vi "Version_2.0_Single_Column_Code.vi"() -> ()   [LabVIEW 2020]
uses:
  C:/Users/Admin/Desktop/MicroPurification/Developer/MainLabViewProject_V2.0/Thorlabs/Thorlabs.MotionControl.Controls.dll
  MainLabViewProject_V2.0/Thorlabs/Thorlabs.MotionControl.Controls.dll
  C:/Users/Admin/Desktop/MicroPurification/Developer/MainLabViewProject_V2.0/Thorlabs/Thorlabs.MotionControl.KCube.InertialMotorCLI.dll
  MainLabViewProject_V2.0/Thorlabs/Thorlabs.MotionControl.KCube.InertialMotorCLI.dll
  <vilib>/Instr/_visa.llb/VISA Configure Serial Port (Instr).vi
  <vilib>/Waveform/WDTOps.llb/WDT Append Waveforms DBL.vi
  <vilib>/Fluigent/Fluigent SDK/sourceCode/fgt_SDK.lvlib
panel:
  in  "n1":dbl=2.0
  in  "Set - Blotting Time":bool
  in  "Set - Blotting Angle":bool
  in  "Automated Blotting \nand Plunging":bool=TRUE
  in  "Blotting Time":dbl=1000.0
  in  "Blotting Angle":dbl=10.0
  in  "Amount of \nGrid Shift \nfor Blotting (um)":i32
  out "Ethane Temperature":dbl
  out "RH (%)":dbl
  out "Valve Closing \nPressure Measured":sgl
  out "Suction pressure \nmeasured":sgl
  in  "Divert Elution Buffer\ninto Column-1":bool
  in  "Discard volume \npriot to elution":dbl=1.0
  in  "Buffer-B Dispense\nFlow Rate for Elution \ntubing pre-wash":dbl=2.0
  in  "Buffer-B Volume \nfor elution tubing \npre-wash":dbl=20.0
  in  "External Valve \nOpen":bool
  in  "N-B1":i32=4
  in  "Valve V10 Open":bool=TRUE
  in  "Valve V9 Open":bool=TRUE
  in  "Valve V8 Open":bool=TRUE
  in  "Capillary purge \nvolume after every\ngrid plunging":dbl=0.05
  in  "Automatic purging \nof capillary after \ngrid deposition":bool=TRUE
  in  "No. of \ncleaning cycles":i32=4
  in  "Pause Elution\nValue":dbl
  in  "Re-SEC":bool
  in  "Buffer-C2 Dispense \nFlow Rate for Washing \nPrior to re-introducing Sample":dbl=2.0
  in  "Buffer-C2 \nWash Volume\nPrior to re-introducing \nSample":dbl=20.0
  in  "Wash column-2 Prior \nto re-introducing \nsample":bool=TRUE
  in  "Valve V7 Open":bool=TRUE
  in  "Valve V6 Open":bool=TRUE
  in  "Valve V5 Open":bool=TRUE
  in  "Fluigent\nLink S/N":u16=10704
  in  "Move Grid \nDown Faster":dbl
  in  "Move Grid \nUp Faster":dbl
  in  "Affinity Elution \nGraph Min CutOff":dbl=1.0
  out "Affinity Elution \nis Approaching":bool
  out "Elution of Column-2":bool
  in  "Port for \nC2-Elution":string="5"
  out "Elution of Column-1":bool
  in  "Port for \nB-Elution":string="7"
  in  "f":dbl
  out "Washing Column-2":bool
  out "Washing Column-1":bool
  in  "Port for \nA2-Wash":string="4"
  out "Sample pumping \ninto Column-1":bool
  out "Equilibriating \nColumn-2":bool
  out "Equilibriating \nColumn-1":bool
  in  "V-S":dbl=10.0
  in  "Port for \nSample":string="3"
  in  "N-S":i32=1
  in  "External Valve \nCLOSED":string="2"
  in  "External Valve \nOPEN":string="1"
  in  "Port for \nC1-Equilibriation":string="5"
  in  "Port for \nA1-Equilibriation":string="4"
  in  "Port-<n> to be \nCleaned (4-9)":i32(ring) items=["4", "5", "6", "7", "8", "9"]
  in  "Clean the \nBuffer-C2 tubing":bool
  in  "Clean the \nBuffer-B tubing":bool=TRUE
  in  "Signal":bool
  out "Net Elution \nVolume":dbl
  out "Pause Elution":bool
  in  "Apparent Volume\nof Syringe":dbl=20.0
  in  "N-C1":i32=4
  in  "N-A1":i32=4
  in  "On-Chip Valve \nClosing\nPressure (mbar)":dbl=1200.0
  in  "Wait time for\ntranslation":u32=100
  out "Suction pressure \nfor grid deposition":sgl
  in  "Suction Pressure\nfor EM-grid \nDeposition (mbar)":sgl
  out "Amplified Signal with Fluid Volume for Affinity Elution":cluster{"Array":dbl[], "Array":dbl[]}(graph)
  out "Affinity Elution On":bool
  out "Amplified Signal with Fluid Volume Near Affinity Elution":cluster{"Array":dbl[], "Array":dbl[]}(graph)
  in  "Valve V4 Open":bool=TRUE
  out "Affinity On":bool
  out "Amplified Signal with Fluid Volume for SEC":cluster{"Array":dbl[], "Array":dbl[]}(graph)
  out "SEC On":bool
  in  "n":i32
  in  "c":dbl
  in  "Duration for \nup/down\nMovement of Grid":u32=100
  in  "Wait time before \nsolenoid for V2\nturns on 2":u32
  in  "Discard Volume":dbl
  out "Discard fluid \nprior to 1st \ndeposition":bool
  in  "Grid Deposition\nDuration":u32
  in  "Valve V3 Open":bool=TRUE
  in  "Valve V2 Open":bool=TRUE
  in  "Valve V1 Open":bool=TRUE
  in  "Delay before\n1st movement\nof grid":dbl
  in  "No of cycles\nof up-down\nmovement":dbl=7.0
  in  "Translation Step SIze\nwhile plunging":dbl=400.0
  in  "Move\nGrid Down":dbl
  in  "Move\nGrid Up":dbl
  in  "k2":dbl
  in  "k1":dbl
  in  "KCubeInertialMotorControl":refnum<k24>(container)
  in  "Select the Action":T1(ring)
  out "Temperature of Ethane Graph":waveform(dbl)(graph)
  in  "Position":i32
  out "True Volume being \ninjected in this\nprocess":dbl
  in  "Buffer-C Volume \nto be Pumped for\nColumn \nnon-interference":dbl
  in  "Buffer-C1 Dispense\nFlow Rate (ul/min) \nfor Equilibration\nof Column-2":dbl=2.0
  in  "Buffer-C1 Volume \nto be  Pumped \nfor Equilibration\nof Column-2":dbl=55.0
  in  "Buffer-C1 Pumping\nResolution \nfor Equilibration \nof Column-2":T2(ring)=enum."High Resolution Pumping"
  in  "Buffer-C1 PickUp \nFlow Rate (ul/min)\nfor Equilibration \nof Column-2":dbl=150.0
  in  "Buffer-A1 Dispense\nFlow Rate (ul/min) \nfor Equilibration\nof Column-1":dbl=2.0
  in  "Buffer-A1 Volume \nto be  Pumped \nfor Equilibration\nof Column-1":dbl=35.0
  in  "Buffer-A1 Pumping\nResolution \nfor Equilibration \nof Column-1":T2(ring)=enum."High Resolution Pumping"
  in  "Buffer-A1 PickUp \nFlow Rate (ul/min)\nfor Equilibration \nof Column-1":dbl=150.0
  out "Buffer-C Volume\nleft to be Pumped":dbl
  in  "Re-deposit Sample\nonto Grid":bool
  in  "Suction On/Off":bool
  out "Vol_previous":dbl
  out "Vol_now":dbl
  out "Position\nNow":dbl
  out "Sample Volume Diverted\ninto Column-2":dbl
  out "Reminder of the \nVolume to be \nPumped":dbl
  in  "Divert Buffer-C \ninto Column-2":bool=TRUE
  in  "Divert Sample \ninto Column-2":bool
  in  "Buffer-B Volume \nto be Pumped for\nSample Diversion\nto Column-2":dbl=0.5
  out "Amplified Signal with Fluid Volume":cluster{"Array":dbl[], "Array":dbl[]}(graph)
  in  "Stop for End of \nExperiment \nand Data Writing":bool
  in  "Select a Process":T3(ring)
  out "Initial Plunger Position":dbl
  out "Stopper that ends \nthe main loops":bool
  in  "Pause /Continue":bool
  in  "Start the Process":bool
  out "Pause Data Collection":bool
  out "Volume being Injected \ntill the end of previous \nprocess":dbl
  out "Total Volume \nbeing Injected":dbl
  out "Volume being Injected \nin this process":dbl
  in  "Divert Sample \nonto Grid":bool=TRUE
  in  "VISA Refnum in\nfor Valve":refnum<visa-resource-name>="COM3"
  in  "Buffer-C2 Dispense\nFlow Rate (ul/min)":dbl=0.25
  in  "Buffer-C2 Volume \nto be Pumped":dbl
  in  "Buffer-C2 Pumping\nResolution":T2(ring)=enum."High Resolution Pumping"
  in  "Buffer-C2 PickUp \nFlow Rate (ul/min)":dbl=150.0
  in  "Buffer-B Dispense\nFlow Rate (ul/min)":dbl=0.25
  in  "Buffer-B Volume \nto be  Pumped":dbl
  in  "Buffer-B Pumping\nResolution":T2(ring)=enum."High Resolution Pumping"
  in  "Buffer-B PickUp \nFlow Rate (ul/min)":dbl=150.0
  in  "Sample Dispense\nFlow Rate (ul/min)":dbl=2.0
  in  "Sample Volume \nto be Pumped":dbl
  in  "Sample Pumping\nResolution":T2(ring)=enum."High Resolution Pumping"
  in  "Sample PickUp \nFlow Rate (ul/min)":dbl=15.0
  in  "Buffer-A2 Dispense\nFlow Rate (ul/min)":dbl=2.0
  in  "Buffer-A2 Volume \nto be Pumped":dbl
  in  "Buffer-A2 Pumping\nResolution":T2(ring)=enum."High Resolution Pumping"
  in  "Buffer-A2 PickUp \nFlow Rate (ul/min)":dbl=150.0
  in  "Volume of Syringe":dbl=25.0
  in  "VISA Refnum in\nfor Pump":refnum<visa-resource-name>="COM4"
  # "More Notes:\n\n- At the start of the experiment, ensure the extrenal valve is detected by teh program\\\n            - Manually unplug and replug the power connection to the valve (locatd near the valve)\n            - Start the program and click on 'Initialize only the valve\" and click on \"Start the Process\"\n            \n\n              - If the program doesn't initialize the valve in 30 sec, turn off the program.\n             -  Manually unplug and replug the power connection to the valve (locatd near the valve) again\n             - Start the LSPone quick softwar on teh desktop and click on the Mnual setting\n             - Choose 'COM3'\n             - Click on Initialize. If teh initialization is sucessful, close this isftware and turn on the \n                 Labview program and try to inialize teh valve. If the valve gets initialized, you are \n                  good to go and use the program further, else redo the process.\n\n- After the above step, while cleaning the tubings\n             - First cleaning ttubings using IPA ....The code is 'clean tubings 3,4, 5and 7\n             - Clean the tubing that goes to teh chip affinity column twice using IPA, run Buffer-A2 pumping code\n             - Clean the tubing that goes to teh chip SEC column twice using IPA, run Buffer-C2 pumping code\n              - Run the above 3 steps with IPA again. This ensures we have teh least bubbles in teh sysetm\n              - Run the 1st 3 steps with water.\n              - After inserting the tubings to the chip, clean teh affinity and SEC columns at 2 ul/min of 30 ul each with water\n              - Before teh start of the main experimnet, run the  code 'clean the tubing from port-3 vial' with Buffer-A once\n\n               - Place teh sample and all teh buffers in the appropriate places and run teh code  with Re-SEC possibility with \n                  appropriate parameters"
  # "Clean only 3,4,5 and 7 \nfor Complex-I\nunless other ports are used"
  # "Notes specific for this code:\n\n- V1 is teh valve just prior to and after affinity column, all other valves are numbered \nclockwise with valve V8 to be teh valve conncecting affinity inlet to waste outlet-2.\n\n- V9 and V10 are valves for affinity wash and elution inlets. Currently they are not used \nin this code.\n\n- Port-8 is connected to the tubing of elution that is conncetcted to column-1 of chip"
  # "Pump Port No           Function\n         1                       Pump Waste\n         2                       Chip Column-1 Connection\n         3                       Sample\n         4                       Buffer- A1 for Equilibriation of Column-1\n         5                       Buffer- C1 for Equilibriation of Column-2\n         6                       Buffer- A2 for Wash of Column-1\n         7                       Buffer- B for Elution of Column-1\n         8                       Buffer-C2 for Elution of Column-2\n         9                       Buffer- A3 for Wash of Column-1\n        10                      Chip Column-2 Connection"
  # "Column-2 Wash Parameters"
  # "Notes:\n- This code uses USB6002 data acquisition device from NI\n- No PGA and only AD8611ARZ preamp\n- Still uses Arduino Uno and Stepper motor \n- Even though designed for Complex-I, but is more generic\n- The code is meant for a chip with 7-onchip valves that are being \ncontrolled using fluigent P-switch, one external on/off valve\nand the pump with 10 ports\n- The tubings \n            - 0.18 mm ID tubings from port-2 to chip, port-3 to sample vial, \nport-10 to SEC inlet of the chip, port-1 to pump-waste\n             - 0.5 mm ID tubings from port-4 to Buffer-A vial, port-5 to \nBuffer-C vial, and port-7 to Buffer-B vial"
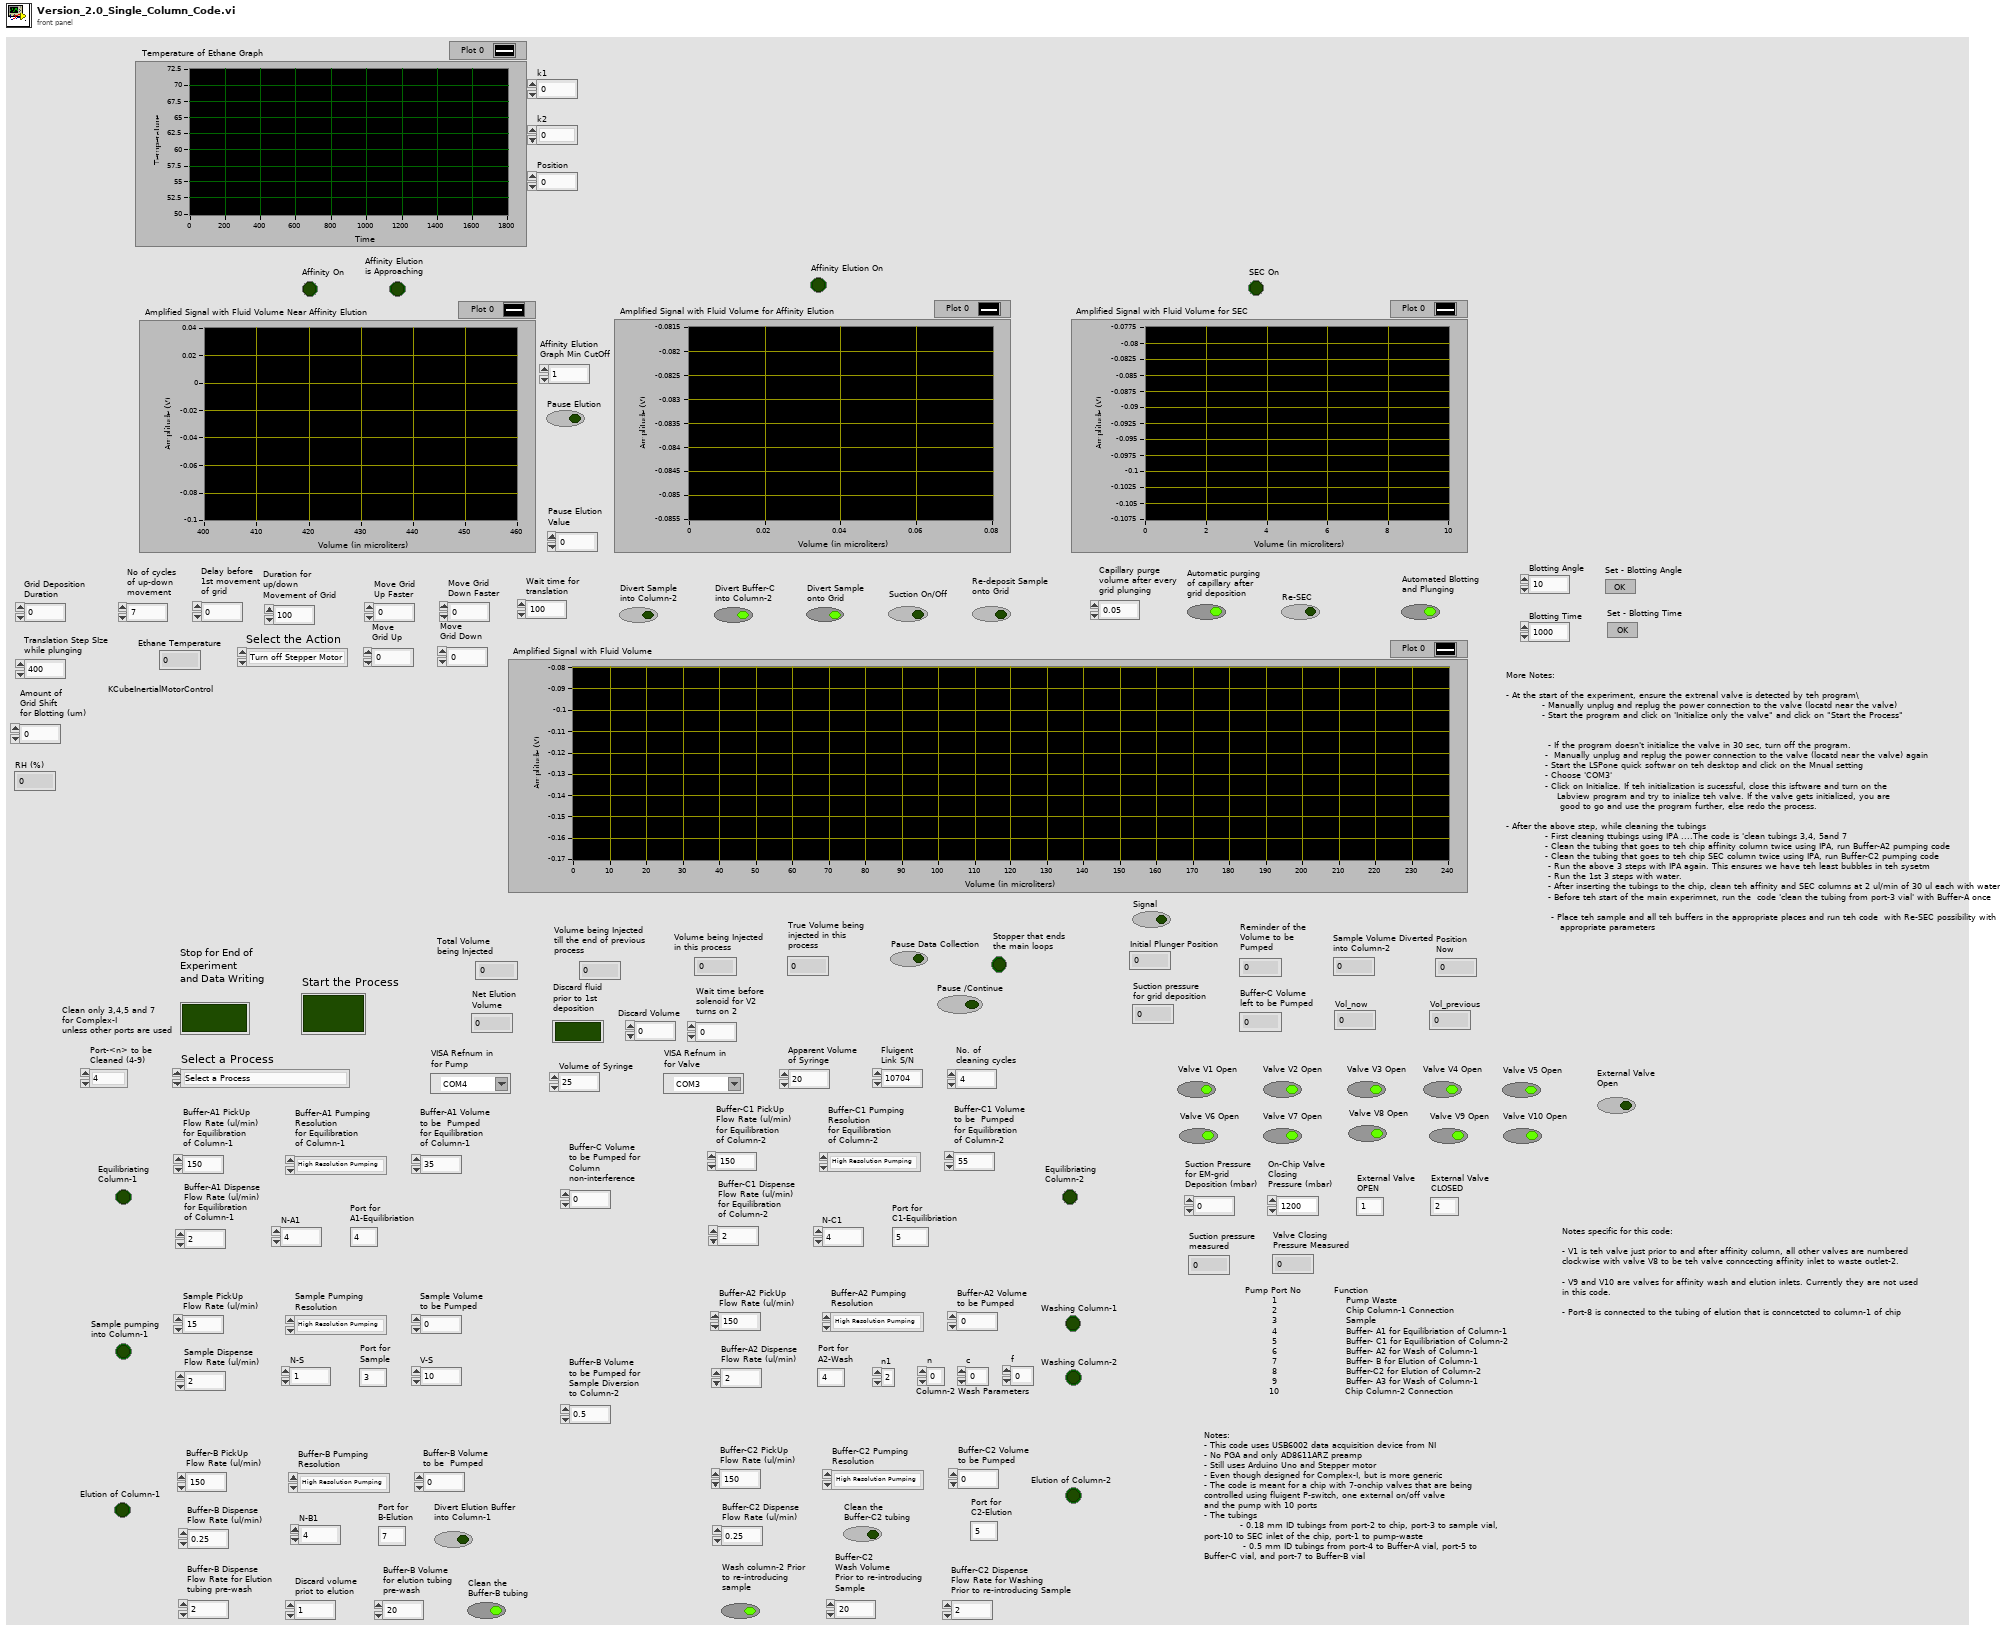
[diagram p1: front panel]
types:
  T1 = enum16{"Turn off Stepper Motor", "Turn  on Stepper Motor", "Spread the deposited protein on the grid in One Line and plunge", "Spread the deposited protein on the grid and plunge", "Start Plunging", "Reset Plunger"}
  T2 = enum16{"Standard Pumping", "High Resolution Pumping"}
  T3 = enum16{"Select a Process", "Initialize Only The Pump", "Initialize Only the Valve", "Initialize Pump and Valve", "Clean the tubing from Port-3 Vial", "Clean the tubing from Port-<n> Vial", "Clean the tubing from Ports 3,4,7 and wash the column", "Clean the tubing from Ports 3,4,5 and 7", "Single Column Automated Protein Purification and Plunging", "Automated Protein Purification with Re-SEC Possibility, 8 SOD Valves and On/Off External Valve", "Automated Protein Purification with 7 SOD Valves and On/Off External Valve", "Automated Plunging Alone Using Purified Protein Via Chip", "Automated Plunging alone using purified protein from SEC column", "Inject Buffer A2, Column 1 with 4 SOD Valves", "Single Column Wash Buffer-A", "Single Column Elution Buffer-B", "Inject Sample, Column 1", "Inject Buffer B, Column 1 with 4 SOD Valves", "Inject Buffer C2, Column 2 with 4 SOD Valves", "Check_Suction_Valve_functionality"}
diagram:
  # "Valve V3 is the on-chip SOD Valve that is after the column-2, after valve V1 and on the way to the waste outlet"
  # "Valve V2 is the on-chip SOD Valve that is after the column-2, after valve V1 and on the way to capillary."
  # "Valve V1 is the on-chip SOD Valve that is after the column-2, just after detection zone-2"
  # "Valve V4 is the on-chip SOD Valve that is after the column-1, just prior to column-2"
  n1 = stacked-sequence {
    frame #0 {
      # "Plunger Control and Ethane Chamber Temperature Display"
      # "AMPLIFIER BLOCK"
      n2 = property class="KCubeInertialMotorControl"(reference="KCubeInertialMotorControl", "SerialNumber"="97102163" ("Serial Number")) -> (reference out=w74:refnum<k24>, error out=w81:errorcluster)  [unwired: 1 in]
      n3 = while {
        stop <- w528 stop-if-true
        n4 = case shown="\"Single Column Automated Protein Purification and Plunging\"" "Select a Process" {
          frame "Initialize Pump and Valve" {
            n5 = local read "Stop for End of \nExperiment \nand Data Writing"() -> (w530:bool)
            n6 = case shown="False" w530 {
              frame False {
                n7 = local read "Start the Process"() -> (w531:bool)
                n8 = case shown="True" w531 {
                  frame False {
                    n9 = local read "Stopper that ends \nthe main loops"() -> (w533:bool)
                    n10 = local read "Start the Process"() -> (w534:bool)
                    n11 = Or(x=w534, y=w533) -> (x .or. y?=w532:bool)
                    n12 = case shown="False" w532 {
                      frame False {
                        n13 = while {
                          stop <- w537 stop-if-true
                          n14 = local read "Stopper that ends \nthe main loops"() -> (w539:bool)
                          n15 = local read "Start the Process"() -> (w538:bool)
                          n16 = Or(x=w538, y=w539) -> (x .or. y?=w537:bool)
                          n17 = Wait (ms)(milliseconds to wait=u32 10) -> ()  [unwired: 1 out]
                        }
                        n18 = One Button Dialog(message="Please select the process and press the 'Start Process' Button") -> ()  [unwired: 1 in, 1 out]
                      }
                      frame True {
                      }
                    }
                  }
                  frame True {
                    n19 = stacked-sequence {
                      frame #0 {
                        n20 = local read "VISA Refnum in\nfor Pump"() -> (w540:refnum<visa-resource-name>)
                        n21 = call "Initializer (SubVI).vi"("VISA Refnum in"=w540) -> ()  [unwired: 11 in]
                      }
                      frame #1 {
                        n22 = local read "VISA Refnum in\nfor Pump"() -> (w541:refnum<visa-resource-name>)
                        n23 = call "ProcessCompletionWaiter (SubVI).vi"("VISA Refnum in"=w541) -> ()  [unwired: 11 in]
                      }
                      frame #2 {
                        n24 = local read "VISA Refnum in\nfor Valve"() -> (w542:refnum<visa-resource-name>)
                        n25 = call "Initializer_Valve (SubVI).vi"("VISA Refnum in"=w542) -> ()  [unwired: 11 in]
                      }
                      frame #3 {
                        n26 = local read "VISA Refnum in\nfor Valve"() -> (w543:refnum<visa-resource-name>)
                        n27 = call "ProcessCompletionWaiter (SubVI).vi"("VISA Refnum in"=w543) -> ()  [unwired: 11 in]
                      }
                      frame #4 {
                        n28 = local write "Start the Process"(FALSE ("Start the Process")) -> ()
                      }
                    }
                  }
                }
              }
              frame True {
              }
            }
          }
          frame "Inject Sample, Column 1" {
            n29 = local read "Stopper that ends \nthe main loops"() -> (w545:bool)
            n30 = case shown="False" w545 {
              frame False {
                n31 = local read "Start the Process"() -> (w546:bool)
                n32 = case shown="True" w546 {
                  frame False {
                    n33 = local read "Stopper that ends \nthe main loops"() -> (w548:bool)
                    n34 = local read "Start the Process"() -> (w547:bool)
                    n35 = Or(x=w548, y=w547) -> (x .or. y?=w549:bool)
                    n36 = case shown="False" w549 {
                      frame False {
                        n37 = while {
                          stop <- w552 stop-if-true
                          n38 = local read "Stopper that ends \nthe main loops"() -> (w554:bool)
                          n39 = local read "Stop for End of \nExperiment \nand Data Writing"() -> (w551:bool)
                          n40 = local read "Start the Process"() -> (w553:bool)
                          n41 = Wait (ms)(milliseconds to wait=u32 10) -> ()  [unwired: 1 out]
                          n42 = Or(x=w554, y=w553) -> (x .or. y?=w552:bool)
                          n43 = local write "Stopper that ends \nthe main loops"(w551) -> ()
                        }
                        n44 = One Button Dialog(message="Please Select the Process and Press 'Start the Process' Button") -> ()  [unwired: 1 in, 1 out]
                      }
                      frame True {
                      }
                    }
                  }
                  frame True {
                    n45 = stacked-sequence {
                      frame #0 {
                        n46 = local read "Sample Volume \nto be Pumped"() -> (w559:dbl)
                        n47 = local read "Apparent Volume\nof Syringe"() -> (w558:dbl)
                        n48 = Quotient & Remainder(x=w559, y=w558) -> (x-y*floor(x/y)=w557:dbl, floor(x/y)=w556:dbl)
                        n49 = for {
                          N: w556 -> [_]
                          n50 = stacked-sequence {
                            frame #0 {
                              # "Switch to Port-3"
                              # "Port-3 of pump is connected to Sample"
                              n51 = local read "VISA Refnum in\nfor Pump"() -> (w561:refnum<visa-resource-name>)
                              n52 = local read "Port for \nSample"() -> (w560:string)
                              n53 = call "PortChanger (SubVI).vi"("Port Number"=w560, "VISA Refnum in"=w561) -> ()  [unwired: 10 in]
                            }
                            frame #1 {
                              n54 = local read "VISA Refnum in\nfor Pump"() -> (w562:refnum<visa-resource-name>)
                              n55 = call "ProcessCompletionWaiter (SubVI).vi"("VISA Refnum in"=w562) -> ()  [unwired: 11 in]
                            }
                            frame #2 {
                              n56 = local read "Sample PickUp \nFlow Rate (ul/min)"() -> (w565:dbl)
                              n57 = local read "Sample Pumping\nResolution"() -> (w564:T2)
                              n58 = local read "VISA Refnum in\nfor Pump"() -> (w567:refnum<visa-resource-name>)
                              n59 = local read "Apparent Volume\nof Syringe"() -> (w563:dbl)
                              n60 = local read "Volume of Syringe"() -> (w566:dbl)
                              n61 = call "RPickUp(SubVI).vi"("Volume to be picked up"=w563, "Volume of Syringe"=w566, "Resolution of PickUP"=w564, "PickUp Flow Rate (ul/min)"=w565, "VISA Refnum in"=w567) -> ()  [unwired: 6 in, 1 out]
                            }
                            frame #3 {
                              n62 = local read "Stopper that ends \nthe main loops"() -> (w568:bool)
                              n63 = local read "VISA Refnum in\nfor Pump"() -> (w569:refnum<visa-resource-name>)
                              n64 = case shown="True" w568 {
                                frame False {
                                }
                                frame True {
                                n65 = local read "VISA Refnum in\nfor Pump"() -> (w570:refnum<visa-resource-name>)
                                n66 = call "HardStopCurrentProcess (SubVI).vi"("VISA Refnum in"=w570) -> ()  [unwired: 11 in]
                                }
                              }
                              n67 = call "ProcessCompletionWaiter (SubVI).vi"("VISA Refnum in"=w569) -> ()  [unwired: 11 in]
                            }
                            frame #4 {
                              # "Reads the initial Plunger Position for computing the volume dispensed"
                              n68 = local read "VISA Refnum in\nfor Pump"() -> (w572:refnum<visa-resource-name>)
                              n69 = call "AbsolutePlungerPosition (SubVI).vi"("VISA Refnum in"=w572) -> ("Plunger Position"=w571:i32)  [unwired: 10 in]
                              n70 = local write "Initial Plunger Position"(w571) -> ()
                            }
                            frame #5 {
                              # "Switch to Port-2"
                              # "Port-2 of the pump is conncted to column-1 of chip"
                              n71 = local read "VISA Refnum in\nfor Pump"() -> (w574:refnum<visa-resource-name>)
                              n72 = call "PortChanger (SubVI).vi"("Port Number"="2", "VISA Refnum in"=w574) -> ()  [unwired: 10 in]
                            }
                            frame #6 {
                              n73 = local read "Stopper that ends \nthe main loops"() -> (w575:bool)
                              n74 = local read "VISA Refnum in\nfor Pump"() -> (w576:refnum<visa-resource-name>)
                              n75 = case shown="True" w575 {
                                frame False {
                                }
                                frame True {
                                n76 = local read "VISA Refnum in\nfor Pump"() -> (w577:refnum<visa-resource-name>)
                                n77 = call "HardStopCurrentProcess (SubVI).vi"("VISA Refnum in"=w577) -> ()  [unwired: 11 in]
                                }
                              }
                              n78 = call "ProcessCompletionWaiter (SubVI).vi"("VISA Refnum in"=w576) -> ()  [unwired: 11 in]
                            }
                            frame #7 {
                              # "Keeps the AMF valve after column-1 open and valve after column-2 closed"
                              n79 = local read "Sample Dispense\nFlow Rate (ul/min)"() -> (w590:dbl)
                              n80 = local read "Sample Pumping\nResolution"() -> (w589:T2)
                              n81 = local read "VISA Refnum in\nfor Pump"() -> (w592:refnum<visa-resource-name>)
                              n82 = local write "Pause Data Collection"(FALSE ("Pause Data Collection")) -> ()
                              n83 = local read "Volume of Syringe"() -> (w591:dbl)
                              n84 = call "GoToAbsolutePosition(SubVI).vi"("Absolute Volume Position in Syringe (in ul)"=0.0 ("Volume to be Dispensed"), "Volume of Syringe"=w591, "Resolution of Pumping"=w589, "Flow Rate (ul/min)"=w590, "VISA Refnum in"=w592) -> ()  [unwired: 6 in, 1 out]
                              n85 = local write "Valve V1 Open"(TRUE ("Valve V1 Open")) -> ()
                              n86 = local write "Valve V2 Open"(TRUE ("Valve V2 Open")) -> ()
                              n87 = local write "Valve V3 Open"(FALSE ("Valve V3 Open")) -> ()
                              n88 = local write "Valve V4 Open"(FALSE ("Valve V4 Open")) -> ()
                              n89 = local write "External Valve \nOpen"(TRUE ("External Valve \nOpen")) -> ()
                              n90 = local write "Valve V8 Open"(FALSE ("Valve V8 Open")) -> ()
                              n91 = local write "Valve V5 Open"(FALSE ("Valve V5 Open")) -> ()
                              n92 = local write "Valve V6 Open"(FALSE ("Valve V6 Open")) -> ()
                              n93 = local write "Valve V7 Open"(FALSE ("Valve V7 Open")) -> ()
                            }
                            frame #8 {
                              n94 = local read "Initial Plunger Position"() -> (w595:dbl)
                              n95 = local read "Sample Pumping\nResolution"() -> (w594:T2)
                              n96 = local read "VISA Refnum in\nfor Pump"() -> (w596:refnum<visa-resource-name>)
                              n97 = local read "Volume of Syringe"() -> (w593:dbl)
                              n98 = stacked-sequence {
                                tunnel: w593 -> [w597]
                                tunnel: w594 -> [w598]
                                tunnel: w595 -> [w600]
                                tunnel: w596 -> [w599]
                                frame #0 {
                                n99 = while {
                                tunnel: w600 -> [w606]
                                tunnel: w599 -> [w605]
                                tunnel: w598 -> [w604]
                                tunnel: w597 -> [w603]
                                stop <- w601 stop-if-true
                                n100 = Wait (ms)(milliseconds to wait=u32 100) -> ()  [unwired: 1 out]
                                n101 = stacked-sequence {
                                tunnel: w606 -> [w612 _]
                                tunnel: w605 -> [w611 w632]
                                tunnel: w604 -> [w610 _]
                                tunnel: w603 -> [w609 _]
                                tunnel: [_ w629] -> w601
                                frame #0 {
                                n102 = call "AbsolutePlungerPosition (SubVI).vi"("VISA Refnum in"=w611) -> ("Plunger Position"=w608:i32)  [unwired: 10 in]
                                n103 = case shown="\"Standard Pumping\", Default" w610 {
                                tunnel: w612 -> [w617 w626]
                                tunnel: w608 -> [w618 w625]
                                tunnel: [w616 w623] -> w607
                                tunnel: w609 -> [w615 w624]
                                frame "Standard Pumping", Default {
                                n104 = Subtract(x=w617, y=w618) -> (x-y=w614:dbl)
                                n105 = Absolute Value(x=w614) -> (abs(x)=w613:dbl)
                                n106 = Multiply(x=w613, y=w615) -> (x*y=w620:dbl)
                                n107 = Divide(x=w620, y=3000.0) -> (x/y=w616:dbl)
                                }
                                frame "High Resolution Pumping" {
                                n108 = Subtract(x=w626, y=w625) -> (x-y=w622:dbl)
                                n109 = Absolute Value(x=w622) -> (abs(x)=w621:dbl)
                                n110 = Multiply(x=w621, y=w624) -> (x*y=w628:dbl)
                                n111 = Divide(x=w628, y=24000.0) -> (x/y=w623:dbl)
                                }
                                }
                                n112 = local write "Volume being Injected \nin this process"(w607) -> ()
                                }
                                frame #1 {
                                n113 = local read "Stopper that ends \nthe main loops"() -> (w631:bool)
                                n114 = call "LSPOneStatus (SubVI).vi"("VISA Refnum in"=w632) -> ("read buffer"=w634:string)  [unwired: 10 in]
                                n115 = call <vilib>:"Trim Whitespace.vi"("string"=w634) -> ("trimmed string"=w633:string)  [unwired: 1 in]
                                n116 = Equal?(x=w633, y="/0`\u0003") -> (x = y?=w630:bool)
                                n117 = Or(x=w630, y=w631) -> (x .or. y?=w629:bool)
                                }
                                }
                                }
                                }
                              }
                            }
                            frame #9 {
                              n118 = local read "Stopper that ends \nthe main loops"() -> (w636:bool)
                              n119 = local write "Pause Data Collection"(TRUE ("Pause Data Collection")) -> ()
                              n120 = local write "Valve V1 Open"(FALSE ("Valve V1 Open")) -> ()
                              n121 = local write "Valve V2 Open"(FALSE ("Valve V2 Open")) -> ()
                              n122 = local write "Valve V3 Open"(FALSE ("Valve V3 Open")) -> ()
                              n123 = local write "Valve V4 Open"(FALSE ("Valve V4 Open")) -> ()
                              n124 = Wait (ms)(milliseconds to wait=u32 500) -> ()  [unwired: 1 out]
                              n125 = case shown="True" w636 {
                                frame False {
                                }
                                frame True {
                                n126 = local read "VISA Refnum in\nfor Pump"() -> (w646:refnum<visa-resource-name>)
                                n127 = call "HardStopCurrentProcess (SubVI).vi"("VISA Refnum in"=w646) -> ()  [unwired: 11 in]
                                }
                              }
                              n128 = local write "Valve V5 Open"(FALSE ("Valve V5 Open")) -> ()
                              n129 = local write "Valve V6 Open"(FALSE ("Valve V6 Open")) -> ()
                              n130 = local write "Valve V7 Open"(FALSE ("Valve V7 Open")) -> ()
                            }
                            frame #10 {
                              n131 = local write "Volume being Injected \nin this process"(0.0 ("Volume being Injected \nin this process")) -> ()
                            }
                          }
                        }
                        n132 = local write "Reminder of the \nVolume to be \nPumped"(w557) -> ()
                      }
                      frame #1 {
                        n133 = stacked-sequence {
                          frame #0 {
                            # "Switch to Port-3"
                            # "Port-3 of pump is connected to Sample"
                            n134 = local read "VISA Refnum in\nfor Pump"() -> (w649:refnum<visa-resource-name>)
                            n135 = local read "Port for \nSample"() -> (w648:string)
                            n136 = call "PortChanger (SubVI).vi"("Port Number"=w648, "VISA Refnum in"=w649) -> ()  [unwired: 10 in]
                          }
                          frame #1 {
                            n137 = local read "VISA Refnum in\nfor Pump"() -> (w650:refnum<visa-resource-name>)
                            n138 = call "ProcessCompletionWaiter (SubVI).vi"("VISA Refnum in"=w650) -> ()  [unwired: 11 in]
                          }
                          frame #2 {
                            n139 = local read "Sample PickUp \nFlow Rate (ul/min)"() -> (w653:dbl)
                            n140 = local read "Sample Pumping\nResolution"() -> (w652:T2)
                            n141 = local read "VISA Refnum in\nfor Pump"() -> (w655:refnum<visa-resource-name>)
                            n142 = local read "Reminder of the \nVolume to be \nPumped"() -> (w651:dbl)
                            n143 = local read "Volume of Syringe"() -> (w654:dbl)
                            n144 = call "RPickUp(SubVI).vi"("Volume to be picked up"=w651, "Volume of Syringe"=w654, "Resolution of PickUP"=w652, "PickUp Flow Rate (ul/min)"=w653, "VISA Refnum in"=w655) -> ()  [unwired: 6 in, 1 out]
                          }
                          frame #3 {
                            n145 = local read "Stopper that ends \nthe main loops"() -> (w656:bool)
                            n146 = local read "VISA Refnum in\nfor Pump"() -> (w657:refnum<visa-resource-name>)
                            n147 = case shown="True" w656 {
                              frame False {
                              }
                              frame True {
                                n148 = local read "VISA Refnum in\nfor Pump"() -> (w658:refnum<visa-resource-name>)
                                n149 = call "HardStopCurrentProcess (SubVI).vi"("VISA Refnum in"=w658) -> ()  [unwired: 11 in]
                              }
                            }
                            n150 = call "ProcessCompletionWaiter (SubVI).vi"("VISA Refnum in"=w657) -> ()  [unwired: 11 in]
                          }
                          frame #4 {
                            # "Reads the initial Plunger Position for computing the volume dispensed"
                            n151 = local read "VISA Refnum in\nfor Pump"() -> (w660:refnum<visa-resource-name>)
                            n152 = call "AbsolutePlungerPosition (SubVI).vi"("VISA Refnum in"=w660) -> ("Plunger Position"=w659:i32)  [unwired: 10 in]
                            n153 = local write "Initial Plunger Position"(w659) -> ()
                          }
                          frame #5 {
                            # "Switch to Port-2"
                            # "Port-2 of the pump is conncted to column-1 of chip"
                            n154 = local read "VISA Refnum in\nfor Pump"() -> (w662:refnum<visa-resource-name>)
                            n155 = call "PortChanger (SubVI).vi"("Port Number"="2", "VISA Refnum in"=w662) -> ()  [unwired: 10 in]
                          }
                          frame #6 {
                            n156 = local read "Stopper that ends \nthe main loops"() -> (w663:bool)
                            n157 = local read "VISA Refnum in\nfor Pump"() -> (w664:refnum<visa-resource-name>)
                            n158 = case shown="True" w663 {
                              frame False {
                              }
                              frame True {
                                n159 = local read "VISA Refnum in\nfor Pump"() -> (w665:refnum<visa-resource-name>)
                                n160 = call "HardStopCurrentProcess (SubVI).vi"("VISA Refnum in"=w665) -> ()  [unwired: 11 in]
                              }
                            }
                            n161 = call "ProcessCompletionWaiter (SubVI).vi"("VISA Refnum in"=w664) -> ()  [unwired: 11 in]
                          }
                          frame #7 {
                            # "Keeps the AMF valve after column-1 open and valve after column-2 closed"
                            n162 = local read "Sample Dispense\nFlow Rate (ul/min)"() -> (w678:dbl)
                            n163 = local read "Sample Pumping\nResolution"() -> (w677:T2)
                            n164 = local read "VISA Refnum in\nfor Pump"() -> (w680:refnum<visa-resource-name>)
                            n165 = local write "Pause Data Collection"(FALSE ("Pause Data Collection")) -> ()
                            n166 = local read "Volume of Syringe"() -> (w679:dbl)
                            n167 = call "GoToAbsolutePosition(SubVI).vi"("Absolute Volume Position in Syringe (in ul)"=0.0 ("Volume to be Dispensed"), "Volume of Syringe"=w679, "Resolution of Pumping"=w677, "Flow Rate (ul/min)"=w678, "VISA Refnum in"=w680) -> ()  [unwired: 6 in, 1 out]
                            n168 = local write "Valve V1 Open"(TRUE ("Valve V1 Open")) -> ()
                            n169 = local write "Valve V2 Open"(TRUE ("Valve V2 Open")) -> ()
                            n170 = local write "Valve V3 Open"(FALSE ("Valve V3 Open")) -> ()
                            n171 = local write "Valve V4 Open"(FALSE ("Valve V4 Open")) -> ()
                            n172 = local write "External Valve \nOpen"(TRUE ("External Valve \nOpen")) -> ()
                            n173 = local write "Valve V5 Open"(FALSE ("Valve V5 Open")) -> ()
                            n174 = local write "Valve V6 Open"(FALSE ("Valve V6 Open")) -> ()
                            n175 = local write "Valve V7 Open"(FALSE ("Valve V7 Open")) -> ()
                            n176 = local write "Valve V8 Open"(FALSE ("Valve V8 Open")) -> ()
                          }
                          frame #8 {
                            n177 = local read "Initial Plunger Position"() -> (w683:dbl)
                            n178 = local read "Sample Pumping\nResolution"() -> (w682:T2)
                            n179 = local read "VISA Refnum in\nfor Pump"() -> (w684:refnum<visa-resource-name>)
                            n180 = local read "Volume of Syringe"() -> (w681:dbl)
                            n181 = stacked-sequence {
                              tunnel: w681 -> [w685]
                              tunnel: w682 -> [w686]
                              tunnel: w683 -> [w688]
                              tunnel: w684 -> [w687]
                              frame #0 {
                                n182 = while {
                                tunnel: w688 -> [w694]
                                tunnel: w687 -> [w693]
                                tunnel: w686 -> [w692]
                                tunnel: w685 -> [w691]
                                stop <- w689 stop-if-true
                                n183 = Wait (ms)(milliseconds to wait=u32 100) -> ()  [unwired: 1 out]
                                n184 = stacked-sequence {
                                tunnel: w694 -> [w700 _]
                                tunnel: w693 -> [w699 w720]
                                tunnel: w692 -> [w698 _]
                                tunnel: w691 -> [w697 _]
                                tunnel: [_ w717] -> w689
                                frame #0 {
                                n185 = call "AbsolutePlungerPosition (SubVI).vi"("VISA Refnum in"=w699) -> ("Plunger Position"=w696:i32)  [unwired: 10 in]
                                n186 = case shown="\"Standard Pumping\", Default" w698 {
                                tunnel: w700 -> [w705 w714]
                                tunnel: w696 -> [w706 w713]
                                tunnel: [w704 w711] -> w695
                                tunnel: w697 -> [w703 w712]
                                frame "Standard Pumping", Default {
                                n187 = Subtract(x=w705, y=w706) -> (x-y=w702:dbl)
                                n188 = Absolute Value(x=w702) -> (abs(x)=w701:dbl)
                                n189 = Multiply(x=w701, y=w703) -> (x*y=w708:dbl)
                                n190 = Divide(x=w708, y=3000.0) -> (x/y=w704:dbl)
                                }
                                frame "High Resolution Pumping" {
                                n191 = Subtract(x=w714, y=w713) -> (x-y=w710:dbl)
                                n192 = Absolute Value(x=w710) -> (abs(x)=w709:dbl)
                                n193 = Multiply(x=w709, y=w712) -> (x*y=w716:dbl)
                                n194 = Divide(x=w716, y=24000.0) -> (x/y=w711:dbl)
                                }
                                }
                                n195 = local write "Volume being Injected \nin this process"(w695) -> ()
                                }
                                frame #1 {
                                n196 = local read "Stopper that ends \nthe main loops"() -> (w719:bool)
                                n197 = call "LSPOneStatus (SubVI).vi"("VISA Refnum in"=w720) -> ("read buffer"=w722:string)  [unwired: 10 in]
                                n198 = call <vilib>:"Trim Whitespace.vi"("string"=w722) -> ("trimmed string"=w721:string)  [unwired: 1 in]
                                n199 = Equal?(x=w721, y="/0`\u0003") -> (x = y?=w718:bool)
                                n200 = Or(x=w718, y=w719) -> (x .or. y?=w717:bool)
                                }
                                }
                                }
                              }
                            }
                          }
                          frame #9 {
                            n201 = local read "Stopper that ends \nthe main loops"() -> (w724:bool)
                            n202 = local write "Pause Data Collection"(TRUE ("Pause Data Collection")) -> ()
                            n203 = local write "Start the Process"(FALSE) -> ()
                            n204 = local write "Valve V1 Open"(FALSE ("Valve V1 Open")) -> ()
                            n205 = local write "Valve V2 Open"(FALSE ("Valve V2 Open")) -> ()
                            n206 = local write "Valve V3 Open"(FALSE ("Valve V3 Open")) -> ()
                            n207 = local write "Valve V4 Open"(FALSE ("Valve V4 Open")) -> ()
                            n208 = Wait (ms)(milliseconds to wait=u32 500) -> ()  [unwired: 1 out]
                            n209 = case shown="True" w724 {
                              frame False {
                              }
                              frame True {
                                n210 = local read "VISA Refnum in\nfor Pump"() -> (w735:refnum<visa-resource-name>)
                                n211 = call "HardStopCurrentProcess (SubVI).vi"("VISA Refnum in"=w735) -> ()  [unwired: 11 in]
                              }
                            }
                            n212 = local write "Valve V5 Open"(FALSE ("Valve V5 Open")) -> ()
                            n213 = local write "Valve V6 Open"(FALSE ("Valve V6 Open")) -> ()
                            n214 = local write "Valve V7 Open"(FALSE ("Valve V7 Open")) -> ()
                          }
                          frame #10 {
                            n215 = local write "Volume being Injected \nin this process"(0.0 ("Volume being Injected \nin this process")) -> ()
                          }
                        }
                      }
                    }
                  }
                }
              }
              frame True {
                n216 = local write "Pause Data Collection"(FALSE ("Pause Data Collection")) -> ()
              }
            }
          }
          frame "Select a Process" {
            n217 = local read "Stopper that ends \nthe main loops"() -> (w738:bool)
            n218 = case shown="False" w738 {
              frame False {
                n219 = stacked-sequence {
                  frame #0 {
                    n220 = local write "Pause Data Collection"(TRUE ("Pause Data Collection")) -> ()
                    n221 = local write "Start the Process"(FALSE ("Start the Process")) -> ()
                  }
                  frame #1 {
                    n222 = local read "Stopper that ends \nthe main loops"() -> (w742:bool)
                    n223 = local read "Start the Process"() -> (w743:bool)
                    n224 = Or(x=w743, y=w742) -> (x .or. y?=w741:bool)
                    n225 = case shown="False" w741 {
                      frame False {
                        n226 = while {
                          stop <- w747 stop-if-true
                          n227 = local read "Stopper that ends \nthe main loops"() -> (w748:bool)
                          n228 = local read "Start the Process"() -> (w749:bool)
                          n229 = local read "Stop for End of \nExperiment \nand Data Writing"() -> (w745:bool)
                          n230 = Wait (ms)(milliseconds to wait=u32 10) -> ()  [unwired: 1 out]
                          n231 = Or(x=w749, y=w748) -> (x .or. y?=w747:bool)
                          n232 = local write "Stopper that ends \nthe main loops"(w745) -> ()
                        }
                        n233 = One Button Dialog(message="Please Select the Process and Press the 'Start the Process' Button") -> ()  [unwired: 1 in, 1 out]
                      }
                      frame True {
                      }
                    }
                  }
                }
              }
              frame True {
                n234 = local write "Pause Data Collection"(FALSE ("Pause Data Collection")) -> ()
              }
            }
          }
          frame "Clean the tubing from Port-3 Vial" {
            n235 = local read "Stopper that ends \nthe main loops"() -> (w751:bool)
            n236 = case shown="False" w751 {
              frame False {
                n237 = local read "Start the Process"() -> (w752:bool)
                n238 = case shown="True" w752 {
                  frame False {
                    n239 = local read "Stopper that ends \nthe main loops"() -> (w754:bool)
                    n240 = local read "Start the Process"() -> (w753:bool)
                    n241 = Or(x=w754, y=w753) -> (x .or. y?=w755:bool)
                    n242 = case shown="False" w755 {
                      frame False {
                        n243 = while {
                          stop <- w758 stop-if-true
                          n244 = local read "Stop for End of \nExperiment \nand Data Writing"() -> (w757:bool)
                          n245 = local read "Stopper that ends \nthe main loops"() -> (w760:bool)
                          n246 = local read "Start the Process"() -> (w759:bool)
                          n247 = Wait (ms)(milliseconds to wait=u32 10) -> ()  [unwired: 1 out]
                          n248 = Or(x=w760, y=w759) -> (x .or. y?=w758:bool)
                          n249 = local write "Stopper that ends \nthe main loops"(w757) -> ()
                        }
                        n250 = One Button Dialog(message="Please Select the Process and Press 'Start the Process' Button") -> ()  [unwired: 1 in, 1 out]
                      }
                      frame True {
                      }
                    }
                  }
                  frame True {
                    n251 = stacked-sequence {
                      frame #0 {
                        n252 = for {
                          N: 1 -> [_]
                          n253 = stacked-sequence {
                            frame #0 {
                              # "Switch to Port-3"
                              # "Port-3 of pump is connected to Sample"
                              n254 = local read "VISA Refnum in\nfor Pump"() -> (w765:refnum<visa-resource-name>)
                              n255 = local write "Pause Data Collection"(TRUE ("Pause Data Collection")) -> ()
                              n256 = call "PortChanger (SubVI).vi"("Port Number"="3", "VISA Refnum in"=w765) -> ()  [unwired: 10 in]
                            }
                            frame #1 {
                              n257 = local read "VISA Refnum in\nfor Pump"() -> (w766:refnum<visa-resource-name>)
                              n258 = call "ProcessCompletionWaiter (SubVI).vi"("VISA Refnum in"=w766) -> ()  [unwired: 11 in]
                            }
                            frame #2 {
                              n259 = local read "VISA Refnum in\nfor Pump"() -> (w771:refnum<visa-resource-name>)
                              n260 = local read "Volume of Syringe"() -> (w770:dbl)
                              n261 = call "RPickUp(SubVI).vi"("Volume to be picked up"=10.0, "Volume of Syringe"=w770, "Resolution of PickUP"=T2."Standard Pumping", "PickUp Flow Rate (ul/min)"=15.0, "VISA Refnum in"=w771) -> ()  [unwired: 6 in, 1 out]
                            }
                            frame #3 {
                              n262 = local read "Stopper that ends \nthe main loops"() -> (w772:bool)
                              n263 = local read "VISA Refnum in\nfor Pump"() -> (w773:refnum<visa-resource-name>)
                              n264 = case shown="True" w772 {
                                frame False {
                                }
                                frame True {
                                n265 = local read "VISA Refnum in\nfor Pump"() -> (w774:refnum<visa-resource-name>)
                                n266 = call "HardStopCurrentProcess (SubVI).vi"("VISA Refnum in"=w774) -> ()  [unwired: 11 in]
                                }
                              }
                              n267 = call "ProcessCompletionWaiter (SubVI).vi"("VISA Refnum in"=w773) -> ()  [unwired: 11 in]
                            }
                            frame #4 {
                              # "Switch to Port-1"
                              # "Port-1 of the pump is conncted to Waste"
                              n268 = local read "VISA Refnum in\nfor Pump"() -> (w776:refnum<visa-resource-name>)
                              n269 = call "PortChanger (SubVI).vi"("Port Number"="1", "VISA Refnum in"=w776) -> ()  [unwired: 10 in]
                            }
                            frame #5 {
                              n270 = local read "Stopper that ends \nthe main loops"() -> (w777:bool)
                              n271 = local read "VISA Refnum in\nfor Pump"() -> (w778:refnum<visa-resource-name>)
                              n272 = case shown="True" w777 {
                                frame False {
                                }
                                frame True {
                                n273 = local read "VISA Refnum in\nfor Pump"() -> (w779:refnum<visa-resource-name>)
                                n274 = call "HardStopCurrentProcess (SubVI).vi"("VISA Refnum in"=w779) -> ()  [unwired: 11 in]
                                }
                              }
                              n275 = call "ProcessCompletionWaiter (SubVI).vi"("VISA Refnum in"=w778) -> ()  [unwired: 11 in]
                            }
                            frame #6 {
                              n276 = local read "VISA Refnum in\nfor Pump"() -> (w784:refnum<visa-resource-name>)
                              n277 = local read "Volume of Syringe"() -> (w783:dbl)
                              n278 = call "GoToAbsolutePosition(SubVI).vi"("Absolute Volume Position in Syringe (in ul)"=0.0 ("Volume to be Dispensed"), "Volume of Syringe"=w783, "Resolution of Pumping"=T2."Standard Pumping" ("Resolution for Dispensing"), "Flow Rate (ul/min)"=150.0 ("Dispense Flow Rate (ul/min)"), "VISA Refnum in"=w784) -> ()  [unwired: 6 in, 1 out]
                            }
                            frame #7 {
                              n279 = local read "Stopper that ends \nthe main loops"() -> (w786:bool)
                              n280 = case shown="True" w786 {
                                frame False {
                                }
                                frame True {
                                n281 = local read "VISA Refnum in\nfor Pump"() -> (w787:refnum<visa-resource-name>)
                                n282 = call "HardStopCurrentProcess (SubVI).vi"("VISA Refnum in"=w787) -> ()  [unwired: 11 in]
                                }
                              }
                              n283 = local read "VISA Refnum in\nfor Pump"() -> (w785:refnum<visa-resource-name>)
                              n284 = call "ProcessCompletionWaiter (SubVI).vi"("VISA Refnum in"=w785) -> ()  [unwired: 11 in]
                            }
                          }
                        }
                      }
                      frame #1 {
                        n285 = local write "Start the Process"(FALSE ("Start the Process")) -> ()
                      }
                    }
                  }
                }
              }
              frame True {
                n286 = local write "Pause Data Collection"(FALSE ("Pause Data Collection")) -> ()
              }
            }
          }
          frame "Clean the tubing from Port-<n> Vial" {
            n287 = local read "Stopper that ends \nthe main loops"() -> (w790:bool)
            n288 = case shown="False" w790 {
              frame False {
                n289 = local read "Start the Process"() -> (w791:bool)
                n290 = case shown="True" w791 {
                  frame False {
                    n291 = local read "Stopper that ends \nthe main loops"() -> (w793:bool)
                    n292 = local read "Start the Process"() -> (w792:bool)
                    n293 = Or(x=w793, y=w792) -> (x .or. y?=w794:bool)
                    n294 = case shown="False" w794 {
                      frame False {
                        n295 = while {
                          stop <- w797 stop-if-true
                          n296 = local read "Stopper that ends \nthe main loops"() -> (w799:bool)
                          n297 = local read "Stop for End of \nExperiment \nand Data Writing"() -> (w796:bool)
                          n298 = local read "Start the Process"() -> (w798:bool)
                          n299 = Wait (ms)(milliseconds to wait=u32 10) -> ()  [unwired: 1 out]
                          n300 = Or(x=w799, y=w798) -> (x .or. y?=w797:bool)
                          n301 = local write "Stopper that ends \nthe main loops"(w796) -> ()
                        }
                        n302 = One Button Dialog(message="Please Select the Process and Press 'Start the Process' Button") -> ()  [unwired: 1 in, 1 out]
                      }
                      frame True {
                      }
                    }
                  }
                  frame True {
                    n303 = stacked-sequence {
                      frame #0 {
                        n304 = local read "No. of \ncleaning cycles"() -> (w801:i32)
                        n305 = for {
                          N: w801 -> [_]
                          n306 = stacked-sequence {
                            frame #0 {
                              # "Switch to Port-4"
                              # "Port-4 of pump is connected to Buffer-A"
                              n307 = local read "VISA Refnum in\nfor Pump"() -> (w804:refnum<visa-resource-name>)
                              n308 = property on="Port-<n> to be \nCleaned (4-9)" class="Ring (strict)"() -> ("RingText.Text"=w802:string)  [unwired: 2 in, 2 out]
                              n309 = local write "Pause Data Collection"(TRUE ("Pause Data Collection")) -> ()
                              n310 = call "PortChanger (SubVI).vi"("Port Number"=w802, "VISA Refnum in"=w804) -> ()  [unwired: 10 in]
                            }
                            frame #1 {
                              n311 = local read "VISA Refnum in\nfor Pump"() -> (w805:refnum<visa-resource-name>)
                              n312 = call "ProcessCompletionWaiter (SubVI).vi"("VISA Refnum in"=w805) -> ()  [unwired: 11 in]
                            }
                            frame #2 {
                              n313 = local read "VISA Refnum in\nfor Pump"() -> (w810:refnum<visa-resource-name>)
                              n314 = local read "Apparent Volume\nof Syringe"() -> (w806:dbl)
                              n315 = local read "Volume of Syringe"() -> (w809:dbl)
                              n316 = call "RPickUp(SubVI).vi"("Volume to be picked up"=w806, "Volume of Syringe"=w809, "Resolution of PickUP"=T2."Standard Pumping", "PickUp Flow Rate (ul/min)"=150.0, "VISA Refnum in"=w810) -> ()  [unwired: 6 in, 1 out]
                            }
                            frame #3 {
                              n317 = local read "Stopper that ends \nthe main loops"() -> (w811:bool)
                              n318 = local read "VISA Refnum in\nfor Pump"() -> (w812:refnum<visa-resource-name>)
                              n319 = case shown="True" w811 {
                                frame False {
                                }
                                frame True {
                                n320 = local read "VISA Refnum in\nfor Pump"() -> (w813:refnum<visa-resource-name>)
                                n321 = call "HardStopCurrentProcess (SubVI).vi"("VISA Refnum in"=w813) -> ()  [unwired: 11 in]
                                }
                              }
                              n322 = call "ProcessCompletionWaiter (SubVI).vi"("VISA Refnum in"=w812) -> ()  [unwired: 11 in]
                            }
                            frame #4 {
                              # "Switch to Port-1"
                              # "Port-1 of the pump is conncted to Waste"
                              n323 = local read "VISA Refnum in\nfor Pump"() -> (w815:refnum<visa-resource-name>)
                              n324 = call "PortChanger (SubVI).vi"("Port Number"="1", "VISA Refnum in"=w815) -> ()  [unwired: 10 in]
                            }
                            frame #5 {
                              n325 = local read "Stopper that ends \nthe main loops"() -> (w816:bool)
                              n326 = local read "VISA Refnum in\nfor Pump"() -> (w817:refnum<visa-resource-name>)
                              n327 = case shown="True" w816 {
                                frame False {
                                }
                                frame True {
                                n328 = local read "VISA Refnum in\nfor Pump"() -> (w818:refnum<visa-resource-name>)
                                n329 = call "HardStopCurrentProcess (SubVI).vi"("VISA Refnum in"=w818) -> ()  [unwired: 11 in]
                                }
                              }
                              n330 = call "ProcessCompletionWaiter (SubVI).vi"("VISA Refnum in"=w817) -> ()  [unwired: 11 in]
                            }
                            frame #6 {
                              n331 = local read "VISA Refnum in\nfor Pump"() -> (w823:refnum<visa-resource-name>)
                              n332 = local read "Volume of Syringe"() -> (w822:dbl)
                              n333 = call "GoToAbsolutePosition(SubVI).vi"("Absolute Volume Position in Syringe (in ul)"=0.0 ("Volume to be Dispensed"), "Volume of Syringe"=w822, "Resolution of Pumping"=T2."Standard Pumping" ("Resolution for Dispensing"), "Flow Rate (ul/min)"=150.0 ("Dispense Flow Rate (ul/min)"), "VISA Refnum in"=w823) -> ()  [unwired: 6 in, 1 out]
                            }
                            frame #7 {
                              n334 = local read "Stopper that ends \nthe main loops"() -> (w825:bool)
                              n335 = case shown="True" w825 {
                                frame False {
                                }
                                frame True {
                                n336 = local read "VISA Refnum in\nfor Pump"() -> (w826:refnum<visa-resource-name>)
                                n337 = call "HardStopCurrentProcess (SubVI).vi"("VISA Refnum in"=w826) -> ()  [unwired: 11 in]
                                }
                              }
                              n338 = local read "VISA Refnum in\nfor Pump"() -> (w824:refnum<visa-resource-name>)
                              n339 = call "ProcessCompletionWaiter (SubVI).vi"("VISA Refnum in"=w824) -> ()  [unwired: 11 in]
                            }
                          }
                        }
                      }
                      frame #1 {
                        n340 = local write "Start the Process"(FALSE ("Start the Process")) -> ()
                      }
                    }
                  }
                }
              }
              frame True {
                n341 = local write "Pause Data Collection"(FALSE ("Pause Data Collection")) -> ()
              }
            }
          }
          frame "Initialize Only The Pump" {
            n342 = local read "Stop for End of \nExperiment \nand Data Writing"() -> (w829:bool)
            n343 = case shown="False" w829 {
              frame False {
                n344 = local read "Start the Process"() -> (w830:bool)
                n345 = case shown="True" w830 {
                  frame False {
                    n346 = local read "Stopper that ends \nthe main loops"() -> (w832:bool)
                    n347 = local read "Start the Process"() -> (w833:bool)
                    n348 = Or(x=w833, y=w832) -> (x .or. y?=w831:bool)
                    n349 = case shown="False" w831 {
                      frame False {
                        n350 = while {
                          stop <- w836 stop-if-true
                          n351 = local read "Stopper that ends \nthe main loops"() -> (w838:bool)
                          n352 = local read "Start the Process"() -> (w837:bool)
                          n353 = Or(x=w837, y=w838) -> (x .or. y?=w836:bool)
                          n354 = Wait (ms)(milliseconds to wait=u32 10) -> ()  [unwired: 1 out]
                        }
                        n355 = One Button Dialog(message="Please select the process and press the 'Start Process' Button") -> ()  [unwired: 1 in, 1 out]
                      }
                      frame True {
                      }
                    }
                  }
                  frame True {
                    n356 = stacked-sequence {
                      frame #0 {
                        n357 = local read "VISA Refnum in\nfor Pump"() -> (w839:refnum<visa-resource-name>)
                        n358 = call "Initializer (SubVI).vi"("VISA Refnum in"=w839) -> ()  [unwired: 11 in]
                      }
                      frame #1 {
                        n359 = local read "VISA Refnum in\nfor Pump"() -> (w840:refnum<visa-resource-name>)
                        n360 = call "ProcessCompletionWaiter (SubVI).vi"("VISA Refnum in"=w840) -> ()  [unwired: 11 in]
                      }
                      frame #2 {
                        n361 = local write "Start the Process"(FALSE ("Start the Process")) -> ()
                      }
                    }
                  }
                }
              }
              frame True {
              }
            }
          }
          frame "Automated Protein Purification with 7 SOD Valves and On/Off External Valve" {
            n362 = local read "Stopper that ends \nthe main loops"() -> (w842:bool)
            n363 = case shown="False" w842 {
              frame False {
                n364 = local read "Start the Process"() -> (w843:bool)
                n365 = case shown="True" w843 {
                  frame False {
                    n366 = local read "Stopper that ends \nthe main loops"() -> (w845:bool)
                    n367 = local read "Start the Process"() -> (w844:bool)
                    n368 = Or(x=w845, y=w844) -> (x .or. y?=w846:bool)
                    n369 = case shown="False" w846 {
                      frame False {
                        n370 = while {
                          stop <- w849 stop-if-true
                          n371 = local read "Stop for End of \nExperiment \nand Data Writing"() -> (w848:bool)
                          n372 = local read "Stopper that ends \nthe main loops"() -> (w851:bool)
                          n373 = local read "Start the Process"() -> (w850:bool)
                          n374 = Wait (ms)(milliseconds to wait=u32 10) -> ()  [unwired: 1 out]
                          n375 = Or(x=w851, y=w850) -> (x .or. y?=w849:bool)
                          n376 = local write "Stopper that ends \nthe main loops"(w848) -> ()
                        }
                        n377 = One Button Dialog(message="Please Select the Process and Press 'Start the Process' Button") -> ()  [unwired: 1 in, 1 out]
                      }
                      frame True {
                      }
                    }
                  }
                  frame True {
                    n378 = stacked-sequence {
                      frame #0 {
                        # "Equilibrate Column-1 with Buffer-A obtained from port-4 and pumped via port-2 and Column-2 with Buffer-C obtained from port-4 and pumped onto chip via port-6 onto the chip ...with an initial and inbetween wash of tubings while changing the buffers"
                        n379 = stacked-sequence {
                          frame #0 {
                            n380 = local read "VISA Refnum in\nfor Valve"() -> (w860:refnum<visa-resource-name>)
                            n381 = local read "External Valve \nCLOSED"() -> (w859:string)
                            n382 = local write "Valve V4 Open"(FALSE ("Valve V4 Open")) -> ()
                            n383 = local write "Valve V1 Open"(FALSE ("Valve V1 Open")) -> ()
                            n384 = local write "Valve V2 Open"(FALSE ("Valve V2 Open")) -> ()
                            n385 = local write "Valve V3 Open"(FALSE ("Valve V3 Open")) -> ()
                            n386 = call "PortChanger_Valve (SubVI).vi"("Port Number"=w859, "VISA Refnum in"=w860) -> ()  [unwired: 10 in]
                            n387 = local write "Valve V7 Open"(FALSE ("Valve V7 Open")) -> ()
                            n388 = local write "Valve V5 Open"(FALSE ("Valve V5 Open")) -> ()
                            n389 = local write "Valve V6 Open"(FALSE ("Valve V6 Open")) -> ()
                            n390 = call <vilib>:"fgt init.vi"() -> ("error out"=w855:errorcluster)  [unwired: 11 in]
                            n391 = while {
                              tunnel: w855 -> [w866]
                              tunnel: [w865] -> w854
                              stop <- w869 stop-if-true
                              # "Keeping the valve closing pressure of push pull to zero"
                              n392 = local read "Stop for End of \nExperiment \nand Data Writing"() -> (w870:bool)
                              n393 = local read "Equilibriating \nColumn-1"() -> (w871:bool)
                              n394 = call <vilib>:"fgt set pressure.vi"("error in (no error)"=w866, "pressure"=sgl 0.0 ("order"), "pressureIndex"=1 ("module")) -> ("error out"=w865:errorcluster)  [unwired: 8 in]
                              n395 = Or(x=w871, y=w870) -> (x .or. y?=w869:bool)
                              n396 = Wait (ms)(milliseconds to wait=u32 10) -> ()  [unwired: 1 out]
                            }
                            n397 = call <vilib>:"fgt close.vi"("error in (no error)"=w854) -> ()  [unwired: 10 in, 1 out]
                          }
                          frame #1 {
                            # "Clean the tubing with Buffer-A1"
                            n398 = local read "N-A1"() -> (w873:i32)
                            n399 = for {
                              N: w873 -> [_]
                              n400 = stacked-sequence {
                                frame #0 {
